vi "Set Meas Step Values.vi"(8 "error in (no error)":errorcluster, 11 "SPECAN_IQSLOT in":refnum<class "SPECAN_IQSLOT.lvclass">) -> (0 "error out":errorcluster, 3 "SPECAN_IQSLOT out":refnum<class "SPECAN_IQSLOT.lvclass">)   [LabVIEW 2018, in "SPECAN_IQSLOT.lvlib" / "SPECAN_IQSLOT.lvclass"]
uses:
  SPECAN_IQSLOT.lvclass
  Plugins/Measurement Interface.lvlibp/Measurement Interface.lvclass
  Plugins/TestStand API Tools (TSAT).lvlibp/Step Actions/TSAT Step Actions.lvlib
  C:/Sequence Automation/Plugins/Measurement Interface.lvlibp/Measurement Interface.lvclass
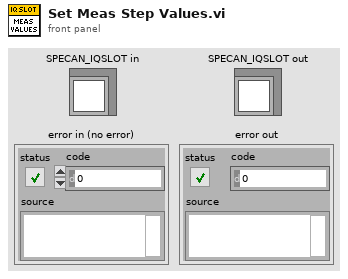
[diagram p1: front panel]
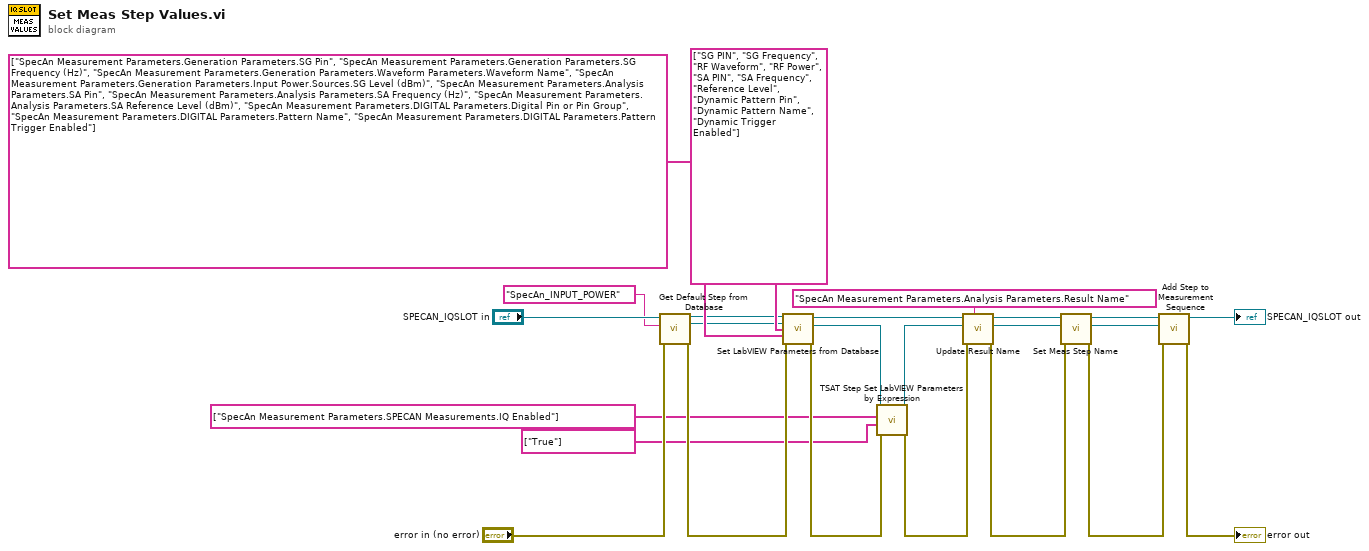
[diagram p0: block diagram]
diagram:
  n1 = call "Get Default Step from Database.vi"("error in (no error)"="error in (no error)", "Default Step"="SpecAn_INPUT_POWER", "Measurement Interface in"="SPECAN_IQSLOT in") -> ("error out"=w13:errorcluster, "Cloned Step"=w15:refnum<k7>, "Measurement Interface out"=w12:refnum<class "SPECAN_IQSLOT.lvclass">)  [unwired: 6 in]
  n2 = call "Set LabVIEW Parameters from Database.vi"("Measurement Interface in"=w12, "Step In"=w15, "Dictionary Keys"=string[] ["SG PIN", "SG Frequency", "RF Waveform", "RF Power", "SA PIN", "SA Frequency", "Reference Level", "Dynamic Pattern Pin", "Dynamic Pattern Name", "Dynamic Trigger Enabled"], "LabVIEW Parameter Mapping"=string[] ["SpecAn Measurement Parameters.Generation Parameters.SG Pin", "SpecAn Measurement Parameters.Generation Parameters.SG Frequency (Hz)", "SpecAn Measurement Parameters.Generation Parameters.Waveform Parameters.Waveform Name", "SpecAn Measurement Parameters.Generation Parameters.Input Power.Sources.SG Level (dBm)", "SpecAn Measurement Parameters.Analysis Parameters.SA Pin", "SpecAn Measurement Parameters.Analysis Parameters.SA Frequency (Hz)", "SpecAn Measurement Parameters.Analysis Parameters.SA Reference Level (dBm)", "SpecAn Measurement Parameters.DIGITAL Parameters.Digital Pin or Pin Group", "SpecAn Measurement Parameters.DIGITAL Parameters.Pattern Name", "SpecAn Measurement Parameters.DIGITAL Parameters.Pattern Trigger Enabled"], "error in (no error)"=w13) -> ("Measurement Interface out"=w6:refnum<class "SPECAN_IQSLOT.lvclass">, "Step Out"=w9:refnum<k7>, "error out"=w21:errorcluster)  [unwired: 8 in]
  n3 = call "TSAT Step Set LabVIEW Parameters by Expression.vi"("Error In"=w21, "Value Expressions"=string[] ["True"], "Parameters to Set"=string[] ["SpecAn Measurement Parameters.SPECAN Measurements.IQ Enabled"], "Step In"=w9) -> ("Error Out"=w22:errorcluster, "Step Out"=w8:refnum<k7>)  [unwired: 6 in]
  n4 = call-dynamic "Update Result Name.vi"("LabVIEW Result Name Parameter"="SpecAn Measurement Parameters.Analysis Parameters.Result Name", "error in (no error)"=w22, "Step In"=w8, "SPECAN_IQSLOT in"=w6) -> ("error out"=w18:errorcluster, "Step Out"=w2:refnum<k7>, "SPECAN_IQSLOT out"=w4:refnum<class "SPECAN_IQSLOT.lvclass">)  [unwired: 5 in]
  n5 = call "Set Meas Step Name.vi"("error in (no error)"=w18, "Step In"=w2, "SPECAN_IQSLOT in"=w4) -> ("error out"=w5:errorcluster, "Step Out"=w1:refnum<k7>, "SPECAN_IQSLOT out"=w3:refnum<class "SPECAN_IQSLOT.lvclass">)  [unwired: 6 in]
  n6 = call "Add Step to Measurement Sequence.vi"("error in (no error)"=w5, "Step to Add"=w1, "Measurement Interface in"=w3) -> ("error out"=→"error out":errorcluster, "Measurement Interface out"=→"SPECAN_IQSLOT out":refnum<class "SPECAN_IQSLOT.lvclass">)  [unwired: 7 in]
